vi "Histogram RT Driver VI.vi"(7 "Operation":T1, 11 "Device Reference in":T2 format="%.0x") -> (0 "Error Code":i32)   [LabVIEW 2012, in "Histogram Custom Device.lvlib"]
uses:
  Histogram Custom Device.lvlib
  <vilib>/NI Veristand/Custom Device API/Custom Device API.lvlib
  <vilib>/NI Veristand/Custom Device API/Custom Device Channel Type.ctl
  <vilib>/NI Veristand/Custom Device API/Data Access Type.ctl
  <vilib>/NI Veristand/Custom Device API/Data Reference.ctl
  BinBounds.ctl
  <vilib>/NI Veristand/Custom Device API/Get Item Property (Variant).vi
  <vilib>/NI Veristand/Custom Device API/Model Interface Driver VI Operation.ctl
  <vilib>/NI Veristand/Custom Device API/Custom Device Item Ref.ctl
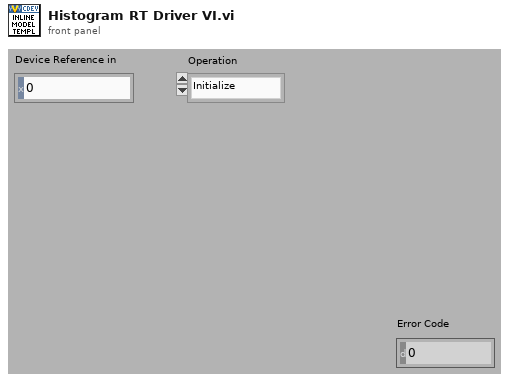
[diagram p1: front panel]
types:
  T1 = typedef "Custom Device API.lvlib/Model Interface Driver VI Operation.ctl" = enum16{"Initialize", "Start", "Execute Model", "Close"}
  T2 = typedef "Custom Device API.lvlib/Custom Device Item Ref.ctl" = u64
  T3 = typedef "Custom Device API.lvlib/Data Reference.ctl" = i32
  T4 = typedef "Histogram Custom Device.lvlib/BinBounds.ctl" = cluster{"Bin Counts":i32[], "Upper Bounds":dbl[], "Lower Bounds":dbl[]}
  T5 = cluster{"Input Values":dbl[], "Input Refs":T3[], "Output Values":dbl[], "Output Refs":T3[], "Cluster":T4}
  T6 = typedef "Custom Device API.lvlib/Custom Device Channel Type.ctl" = enum16{"Input", "Output"}
  T7 = typedef "Custom Device API.lvlib/Data Access Type.ctl" = enum16{"Read", "Write"}
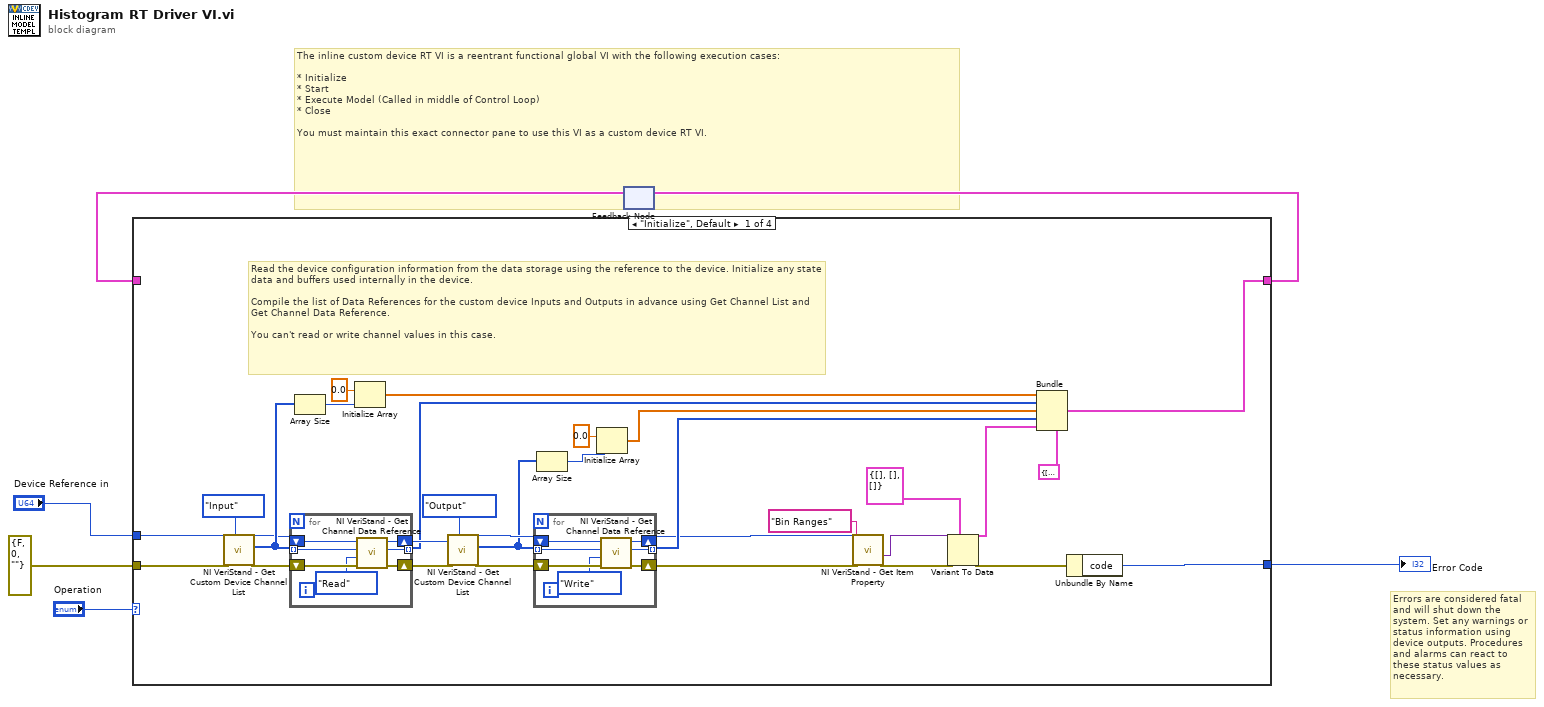
[diagram p0: block diagram]
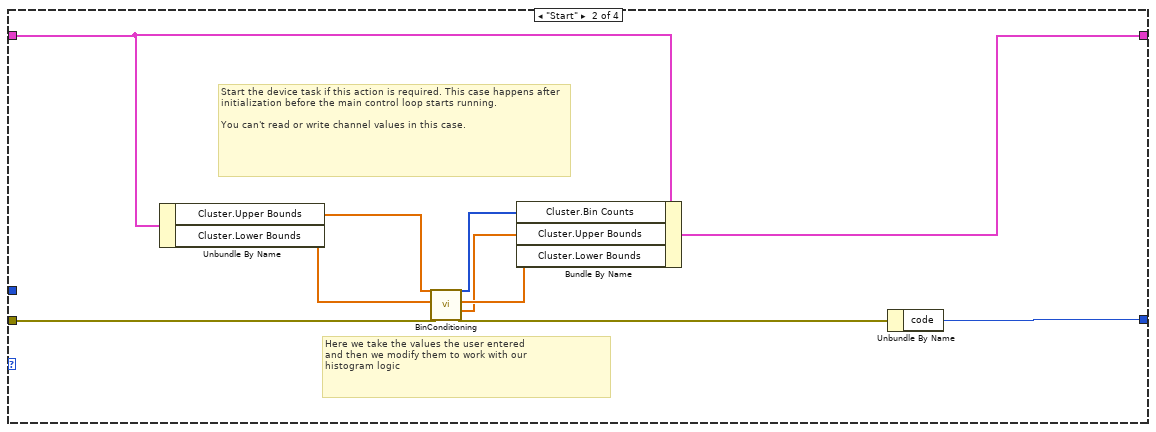
[diagram p2: hidden frame]
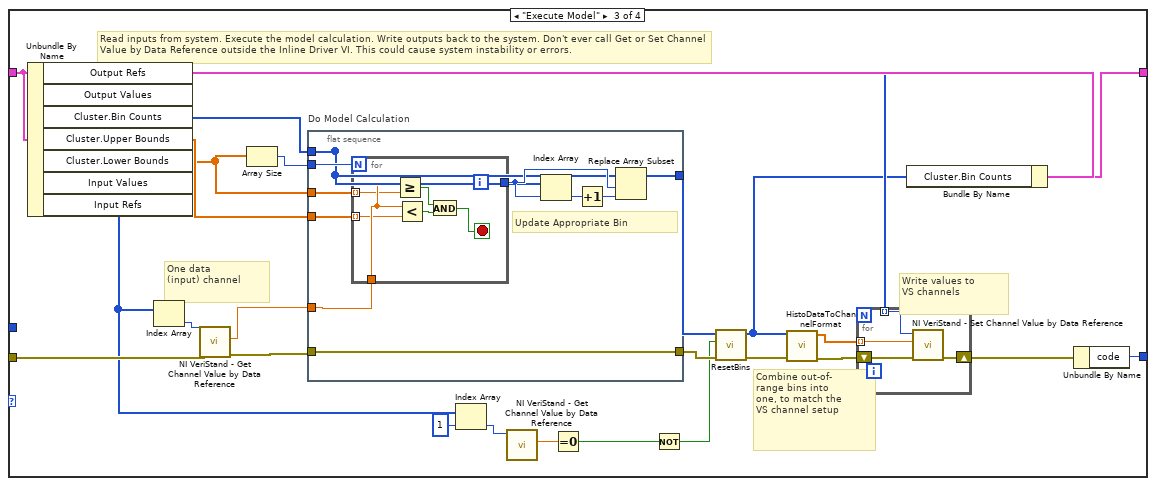
[diagram p3: hidden frame]
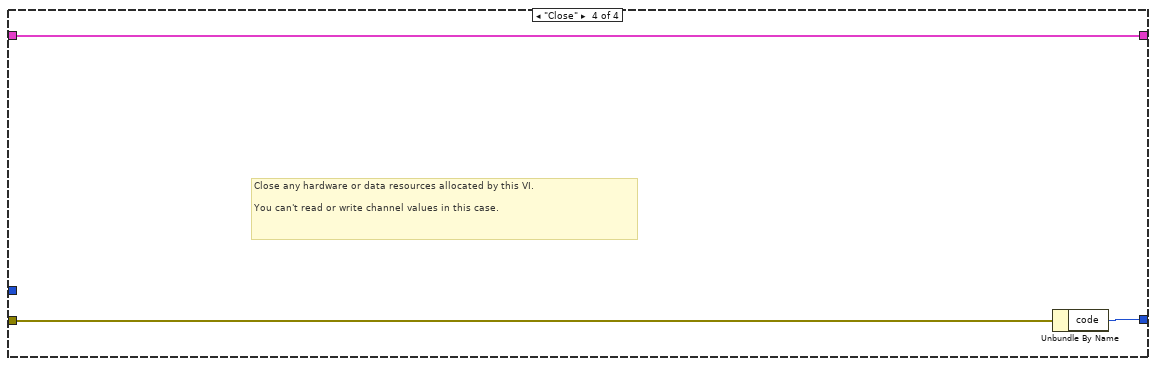
[diagram p4: hidden frame]
diagram:
  # "Errors are considered fatal and will shut down the system. Set any warnings or status information using device outputs. Procedures and alarms can react to these status values as necessary."
  # "The inline custom device RT VI is a reentrant functional global VI with the following execution cases:\n\n* Initialize\n* Start\n* Execute Model (Called in middle of Control Loop)\n* Close\n\nYou must maintain this exact connector pane to use this VI as a custom device RT VI."
  n1 = feedback #1() -> (w4:T5)  [unwired: 1 out]
  n2 = case shown="\"Initialize\", Default" "Operation" {
    tunnel: [w16 w58 w83 w110] -> w5
    tunnel: w4 -> [_ w59 w84 w110]
    tunnel: "Device Reference in" -> [w17 _ _ _]
    tunnel: [w15 w60 w82 w109] -> w2
    tunnel: errorcluster {"status"=FALSE, "code"=0, "source"=""} ("error in (no error)") -> [w14 w61 w86 w108]
    frame "Initialize", Default {
      # "Read the device configuration information from the data storage using the reference to the device. Initialize any state data and buffers used internally in the device.\n\nCompile the list of Data References for the custom device Inputs and Outputs in advance using Get Channel List and Get Channel Data Reference.\n\nYou can't read or write channel values in this case."
      n3 = call <vilib>:"NI VeriStand - Get Custom Device Channel List.vi"("Channel Type"=Custom_Device_Channel_Type."Input", "error in (no error)"=w14, "Device Ref in"=w17) -> ("error out"=w23:errorcluster, "Specified Channel Ref List"=w24:T2[], "Device Ref out"=w22:T2)  [unwired: 6 out]
      n4 = for {
        shift-right: [w46] -> w36
        shift-left: w22 -> [w50]
        tunnel: w24 -> [w49] mode=indexing
        shift-right: [w47] -> w27
        shift-left: w23 -> [w51]
        tunnel: [w45] -> w28 mode=indexing
        n5 = call <vilib>:"NI VeriStand - Get Channel Data Reference.vi"("error in (no error)"=w51, "Access"=Data_Access_Type."Read", "Channel Ref in"=w49, "Device Ref in"=w50) -> ("error out"=w47:errorcluster, "Channel Data Reference"=w45:T3, "Device Ref out"=w46:T2)  [unwired: 5 out]
      }
      n6 = Array Size(array=w24) -> (size(s)=w19:i32)
      n7 = Initialize Array(0.0 ("element"), w19) -> (w18:dbl[])
      n8 = call <vilib>:"NI VeriStand - Get Custom Device Channel List.vi"("Channel Type"=Custom_Device_Channel_Type."Output", "error in (no error)"=w27, "Device Ref in"=w36) -> ("error out"=w25:errorcluster, "Specified Channel Ref List"=w31:T2[], "Device Ref out"=w37:T2)  [unwired: 6 out]
      n9 = for {
        tunnel: w31 -> [w42] mode=indexing
        shift-right: [w40] -> w34
        shift-left: w25 -> [w44]
        tunnel: [w39] -> w33 mode=indexing
        shift-right: [w38] -> w12
        shift-left: w37 -> [w43]
        n10 = call <vilib>:"NI VeriStand - Get Channel Data Reference.vi"("error in (no error)"=w44, "Access"=Data_Access_Type."Write", "Channel Ref in"=w42, "Device Ref in"=w43) -> ("error out"=w40:errorcluster, "Channel Data Reference"=w39:T3, "Device Ref out"=w38:T2)  [unwired: 5 out]
      }
      n11 = Array Size(array=w31) -> (size(s)=w30:i32)
      n12 = Initialize Array(0.0 ("element"), w30) -> (w32:dbl[])
      n13 = call-poly <vilib>:"NI VeriStand - Get Item Property.vi"("error in (no error)"=w34, "Property Name"="Bin Ranges", "Item Ref in"=w12) -> ("error out"=w13:errorcluster, "Value"=w8:variant)  [unwired: 5 in, 2 out]
      n14 = Variant To Data(error in=w13, type=T4 {"Bin Counts"=[], "Upper Bounds"=[], "Lower Bounds"=[]} ("Cluster"), Variant=w8) -> (data=w7:T4, error out=w10:errorcluster)
      n15 = Bundle(cluster=T5 {"Input Values"=[], "Input Refs"=[], "Output Values"=[], "Output Refs"=[], "Cluster"={"Bin Counts"=[], "Upper Bounds"=[], "Lower Bounds"=[]}}, "Input Values"=w18, "Input Refs"=w28, "Output Values"=w32, "Output Refs"=w33, "Cluster"=w7) -> (w16:T5)
      n16 = Unbundle By Name(w10) -> ("code"=w15:i32)
    }
    frame "Start" {
      # "Here we take the values the user entered\nand then we modify them to work with our\nhistogram logic"
      # "Start the device task if this action is required. This case happens after initialization before the main control loop starts running.\n\nYou can't read or write channel values in this case."
      n17 = Unbundle By Name(w59) -> ("Cluster.Upper Bounds"=w56:dbl[], "Cluster.Lower Bounds"=w55:dbl[])
      n18 = call "BinConditioning.vi"("error in (no error)"=w61, "Lower Bounds"=w55, "Upper Bounds"=w56) -> ("error out"=w57:errorcluster, "Upper Bounds"=w52:dbl[], "Lower Bounds"=w53:dbl[], "Bin Counts"=w54:i32[])  [unwired: 5 in]
      n19 = Bundle By Name(cluster=w59, "Cluster.Bin Counts"=w54, "Cluster.Upper Bounds"=w52, "Cluster.Lower Bounds"=w53) -> (w58:T5)
      n20 = Unbundle By Name(w57) -> ("code"=w60:i32)
    }
    frame "Execute Model" {
      # "Write values to \nVS channels"
      # "Combine out-of- \nrange bins into\none, to match the\nVS channel setup"
      # "One data \n(input) channel"
      # "Read inputs from system. Execute the model calculation. Write outputs back to the system. Don't ever call Get or Set Channel Value by Data Reference outside the Inline Driver VI. This could cause system instability or errors."
      n21 = Unbundle By Name(w84) -> ("Output Refs"=w75:T3[], "Cluster.Bin Counts"=w78:i32[], "Cluster.Upper Bounds"=w77:dbl[], "Cluster.Lower Bounds"=w76:dbl[], "Input Refs"=w73:T3[])  [unwired: 2 out]
      n22 = Index Array(array=w73) -> (element=w80:T3)  [unwired: 1 in]
      n23 = call <vilib>:"NI VeriStand - Get Channel Value by Data Reference.vi"("error in (no error)"=w86, "Data Reference in"=w80) -> ("error out"=w85:errorcluster, "Value"=w79:dbl)  [unwired: 8 out]
      n24 = Array Size(array=w76) -> (size(s)=w81:i32)
      n25 = flat-sequence "Do Model Calculation" {
        tunnel: w85 -> [w100]
        tunnel: [w100] -> w74
        tunnel: w81 -> [w99]
        tunnel: w79 -> [w98]
        tunnel: w77 -> [w97]
        tunnel: [w93] -> _
        tunnel: w78 -> [w93]
        tunnel: w76 -> [w92]
        tunnel: [w91] -> w64
        frame #0 {
          # "Update Appropriate Bin"
          n26 = for {
            N: w99 -> [_]
            tunnel: w98 -> [w105]
            tunnel: w97 -> [w104] mode=indexing
            tunnel: [w102] -> w94
            tunnel: w92 -> [w101] mode=indexing
            i -> [w102]
            stop <- w103 stop-if-true
            n27 = Greater Or Equal?(x=w105, y=w101) -> (x >= y?=w106:bool)
            n28 = Less?(x=w105, y=w104) -> (x < y?=w107:bool)
            n29 = And(x=w106, y=w107) -> (x .and. y?=w103:bool)
          }
          n30 = Index Array(array=w93, index=w94) -> (element=w95:i32)
          n31 = Increment(x=w95) -> (x+1=w96:i32)
          n32 = Replace Array Subset(array=w93, new element=w96, index=w94) -> (w91:i32[])
        }
      }
      n33 = Index Array(array=w73, index=1) -> (element=w68:T3)
      n34 = call <vilib>:"NI VeriStand - Get Channel Value by Data Reference.vi"("Data Reference in"=w68) -> ("Value"=w71:dbl)  [unwired: 1 in, 9 out]
      n35 = Equal To 0?(x=w71) -> (x = 0?=w70:bool)
      n36 = Not(x=w70) -> (.not. x?=w62:bool)
      n37 = call "ResetBins.vi"("error in"=w74, "Reset?"=w62, "Channel Data in"=w64) -> ("error out"=w65:errorcluster, "Channel Data out"=w63:i32[])  [unwired: 7 in]
      n38 = call "HistoDataToChannelFormat.vi"("error in"=w65, "Histo Bins"=w63) -> ("error out"=w67:errorcluster, "Channel Data"=w66:dbl[])  [unwired: 8 in]
      n39 = for "Write Output \nValues to System" {
        shift-right: [w89] -> w69
        shift-left: w67 -> [w90]
        tunnel: w75 -> [w88] mode=indexing
        tunnel: w66 -> [w87] mode=indexing
        n40 = call <vilib>:"NI VeriStand - Set Channel Value by Data Reference.vi"("error in (no error)"=w90, "Value"=w87, "Data Reference in"=w88) -> ("error out"=w89:errorcluster)  [unwired: 8 out]
      }
      n41 = Bundle By Name(cluster=w84, "Cluster.Bin Counts"=w63) -> (w83:T5)
      n42 = Unbundle By Name(w69) -> ("code"=w82:i32)
    }
    frame "Close" {
      # "Close any hardware or data resources allocated by this VI.\n\nYou can't read or write channel values in this case."
      n43 = Unbundle By Name(w108) -> ("code"=w109:i32)
    }
  }
  "Error Code" <- w2
  n44 = feedback-in #1(w5) -> ()
